vi "Write grouped data to tags.vi"(9 "Indices":i32[](array[numeric]), 10 "Data Type":T1, 11 "Data":T2) -> ()   [LabVIEW 2016, in "CVT.lvlib" / "Current Value Table.lvlib"]
uses:
  <vilib>/NI/Current Value Table/Current Value Table.lvlib
  <vilib>/NI/Current Value Table/Type Defs/Group Data.ctl
  <vilib>/NI/Current Value Table/Type Defs/Data Types.ctl
  <vilib>/NI/Current Value Table/DataTypes/Double_Write Index Set.vi
  <vilib>/NI/Current Value Table/DataTypes/Array of String_Write Index Set.vi
  <vilib>/NI/Current Value Table/DataTypes/Array of Boolean_Write Index Set.vi
  <vilib>/NI/Current Value Table/DataTypes/Array of Single_Write Index Set.vi
  <vilib>/NI/Current Value Table/DataTypes/Array of Double_Write Index Set.vi
  <vilib>/NI/Current Value Table/DataTypes/Array of I8_Write Index Set.vi
  <vilib>/NI/Current Value Table/DataTypes/Array of I16_Write Index Set.vi
  <vilib>/NI/Current Value Table/DataTypes/Array of I32_Write Index Set.vi
  <vilib>/NI/Current Value Table/DataTypes/Array of I64_Write Index Set.vi
  <vilib>/NI/Current Value Table/DataTypes/Array of U64_Write Index Set.vi
  <vilib>/NI/Current Value Table/DataTypes/Array of U32_Write Index Set.vi
  <vilib>/NI/Current Value Table/DataTypes/Array of U16_Write Index Set.vi
  <vilib>/NI/Current Value Table/DataTypes/Array of U8_Write Index Set.vi
  <vilib>/NI/Current Value Table/DataTypes/Boolean_Write Index Set.vi
  <vilib>/NI/Current Value Table/DataTypes/String_Write Index Set.vi
  <vilib>/NI/Current Value Table/DataTypes/U8_Write Index Set.vi
  <vilib>/NI/Current Value Table/DataTypes/U16_Write Index Set.vi
  <vilib>/NI/Current Value Table/DataTypes/U32_Write Index Set.vi
  <vilib>/NI/Current Value Table/DataTypes/U64_Write Index Set.vi
  <vilib>/NI/Current Value Table/DataTypes/I8_Write Index Set.vi
  <vilib>/NI/Current Value Table/DataTypes/I16_Write Index Set.vi
  <vilib>/NI/Current Value Table/DataTypes/I32_Write Index Set.vi
  <vilib>/NI/Current Value Table/DataTypes/I64_Write Index Set.vi
  <vilib>/NI/Current Value Table/DataTypes/Single_Write Index Set.vi
  <vilib>/NI/Current Value Table/Memory Block.vi
  <vilib>/NI/Current Value Table/DataTypes/Single_Memory Block.vi
  <vilib>/NI/Current Value Table/DataTypes/I64_Memory Block.vi
  <vilib>/NI/Current Value Table/DataTypes/I32_Memory Block.vi
  <vilib>/NI/Current Value Table/DataTypes/I16_Memory Block.vi
  <vilib>/NI/Current Value Table/DataTypes/I8_Memory Block.vi
  <vilib>/NI/Current Value Table/DataTypes/U64_Memory Block.vi
  <vilib>/NI/Current Value Table/DataTypes/U32_Memory Block.vi
  <vilib>/NI/Current Value Table/DataTypes/U16_Memory Block.vi
  <vilib>/NI/Current Value Table/DataTypes/U8_Memory Block.vi
  <vilib>/NI/Current Value Table/DataTypes/String_Memory Block.vi
  <vilib>/NI/Current Value Table/DataTypes/Boolean_Memory Block.vi
  <vilib>/NI/Current Value Table/DataTypes/Array of U8_Memory Block.vi
  <vilib>/NI/Current Value Table/DataTypes/Array of U16_Memory Block.vi
  <vilib>/NI/Current Value Table/DataTypes/Array of U32_Memory Block.vi
  <vilib>/NI/Current Value Table/DataTypes/Array of U64_Memory Block.vi
  <vilib>/NI/Current Value Table/DataTypes/Array of I64_Memory Block.vi
  <vilib>/NI/Current Value Table/DataTypes/Array of I32_Memory Block.vi
  <vilib>/NI/Current Value Table/DataTypes/Array of I16_Memory Block.vi
  <vilib>/NI/Current Value Table/DataTypes/Array of I8_Memory Block.vi
  <vilib>/NI/Current Value Table/DataTypes/Array of Double_Memory Block.vi
  <vilib>/NI/Current Value Table/DataTypes/Array of Single_Memory Block.vi
  <vilib>/NI/Current Value Table/DataTypes/Array of Boolean_Memory Block.vi
  <vilib>/NI/Current Value Table/DataTypes/Array of String_Memory Block.vi
  <vilib>/NI/Current Value Table/DataTypes/Double_Memory Block.vi
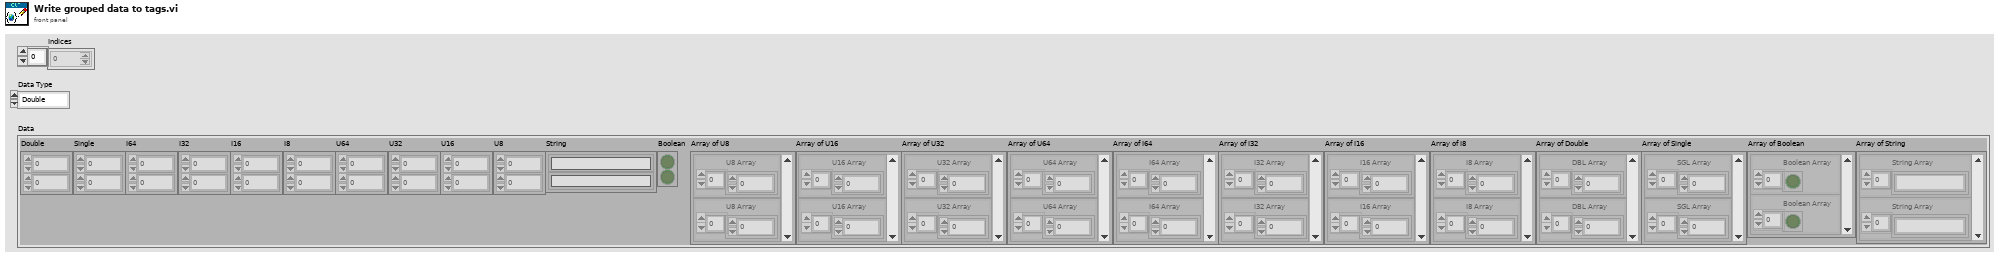
[diagram p1: front panel]
types:
  T1 = typedef "CVT.lvlib/Current Value Table.lvlib/Data Types.ctl" = enum16{"Double", "Single", "I64", "I32", "I16", "I8", "U64", "U32", "U16", "U8", "String", "Boolean", "Array of U8", "Array of U16", "Array of U32", "Array of U64", "Array of I64", "Array of I32", "Array of I16", "Array of I8", "Array of Double", "Array of Single", "Array of Boolean", "Array of String"}
  T2 = typedef "CVT.lvlib/Current Value Table.lvlib/Group Data.ctl" = cluster{"Double":dbl[], "Single":sgl[], "I64":i64[], "I32":i32[], "I16":i16[], "I8":i8[], "U64":u64[], "U32":u32[], "U16":u16[], "U8":u8[], "String":string[], "Boolean":bool[], "Array of U8":cluster{"U8 Array":u8[]}[], "Array of U16":cluster{"U16 Array":u16[]}[], "Array of U32":cluster{"U32 Array":u32[]}[], "Array of U64":cluster{"U64 Array":u64[]}[], "Array of I64":cluster{"I64 Array":i64[]}[], "Array of I32":cluster{"I32 Array":i32[]}[], "Array of I16":cluster{"I16 Array":i16[]}[], "Array of I8":cluster{"I8 Array":i8[]}[], "Array of Double":cluster{"DBL Array":dbl[]}[], "Array of Single":cluster{"SGL Array":sgl[]}[], "Array of Boolean":cluster{"Boolean Array":bool[]}[], "Array of String":cluster{"String Array":string[]}[]}
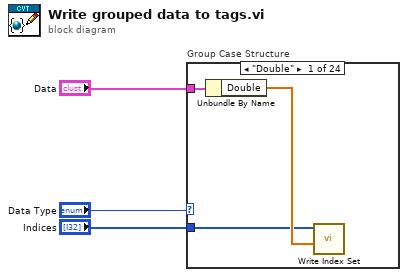
[diagram p0: block diagram]
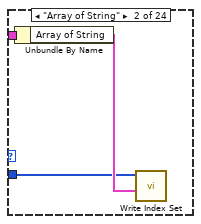
[diagram p2: hidden frame]
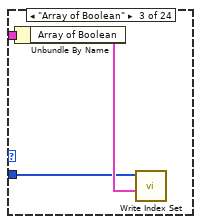
[diagram p3: hidden frame]
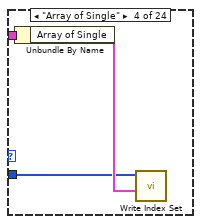
[diagram p4: hidden frame]
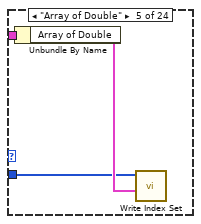
[diagram p5: hidden frame]
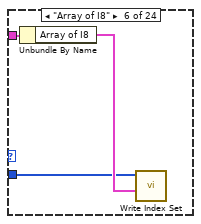
[diagram p6: hidden frame]
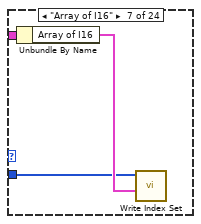
[diagram p7: hidden frame]
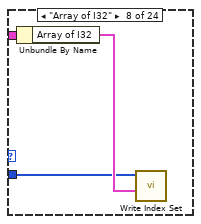
[diagram p8: hidden frame]
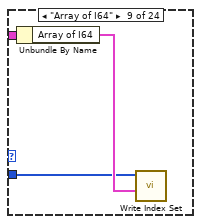
[diagram p9: hidden frame]
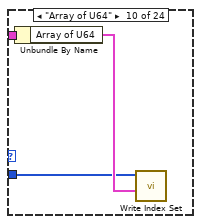
[diagram p10: hidden frame]
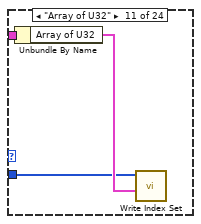
[diagram p11: hidden frame]
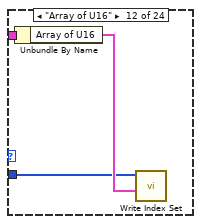
[diagram p12: hidden frame]
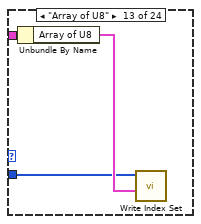
[diagram p13: hidden frame]
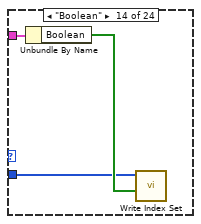
[diagram p14: hidden frame]
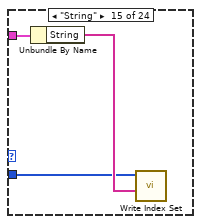
[diagram p15: hidden frame]
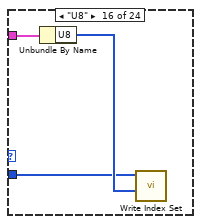
[diagram p16: hidden frame]
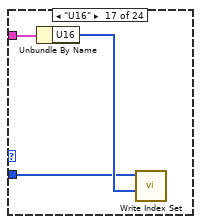
[diagram p17: hidden frame]
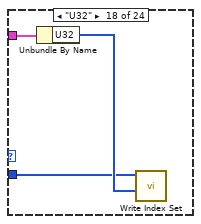
[diagram p18: hidden frame]
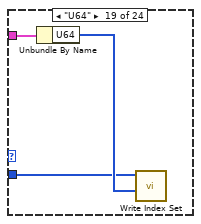
[diagram p19: hidden frame]
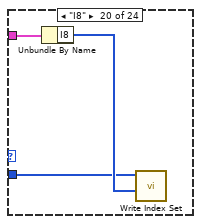
[diagram p20: hidden frame]
diagram:
  n1 = case "Group Case Structure" shown="\"Double\"" "Data Type" {
    tunnel: "Data" -> [w6 w9 w12 w15 w18 w21 w24 w27 w30 w33 w36 w39 w42 w45 w48 w51 w54 w57 w60 w63 w66 w69 w72 w75]
    tunnel: "Indices" -> [w4 w7 w10 w13 w16 w19 w22 w25 w28 w31 w34 w37 w40 w43 w46 w49 w52 w55 w58 w61 w64 w67 w70 w73]
    frame "Double" {
      n2 = Unbundle By Name(w6) -> ("Double"=w5:dbl[])
      n3 = call-poly <vilib>:"Write Index Set.vi"("Values"=w5, "Indices"=w4) -> ()  [unwired: 10 in]
    }
    frame "Array of String" {
      n4 = Unbundle By Name(w9) -> ("Array of String"=w8:cluster{"String Array":string[]}[])
      n5 = call-poly <vilib>:"Write Index Set.vi"("Values"=w8, "Indices"=w7) -> ()  [unwired: 10 in]
    }
    frame "Array of Boolean" {
      n6 = Unbundle By Name(w12) -> ("Array of Boolean"=w11:cluster{"Boolean Array":bool[]}[])
      n7 = call-poly <vilib>:"Write Index Set.vi"("Values"=w11, "Indices"=w10) -> ()  [unwired: 10 in]
    }
    frame "Array of Single" {
      n8 = Unbundle By Name(w15) -> ("Array of Single"=w14:cluster{"SGL Array":sgl[]}[])
      n9 = call-poly <vilib>:"Write Index Set.vi"("Values"=w14, "Indices"=w13) -> ()  [unwired: 10 in]
    }
    frame "Array of Double" {
      n10 = Unbundle By Name(w18) -> ("Array of Double"=w17:cluster{"DBL Array":dbl[]}[])
      n11 = call-poly <vilib>:"Write Index Set.vi"("Values"=w17, "Indices"=w16) -> ()  [unwired: 10 in]
    }
    frame "Array of I8" {
      n12 = Unbundle By Name(w21) -> ("Array of I8"=w20:cluster{"I8 Array":i8[]}[])
      n13 = call-poly <vilib>:"Write Index Set.vi"("Values"=w20, "Indices"=w19) -> ()  [unwired: 10 in]
    }
    frame "Array of I16" {
      n14 = Unbundle By Name(w24) -> ("Array of I16"=w23:cluster{"I16 Array":i16[]}[])
      n15 = call-poly <vilib>:"Write Index Set.vi"("Values"=w23, "Indices"=w22) -> ()  [unwired: 10 in]
    }
    frame "Array of I32" {
      n16 = Unbundle By Name(w27) -> ("Array of I32"=w26:cluster{"I32 Array":i32[]}[])
      n17 = call-poly <vilib>:"Write Index Set.vi"("Values"=w26, "Indices"=w25) -> ()  [unwired: 10 in]
    }
    frame "Array of I64" {
      n18 = Unbundle By Name(w30) -> ("Array of I64"=w29:cluster{"I64 Array":i64[]}[])
      n19 = call-poly <vilib>:"Write Index Set.vi"("Values"=w29, "Indices"=w28) -> ()  [unwired: 10 in]
    }
    frame "Array of U64" {
      n20 = Unbundle By Name(w33) -> ("Array of U64"=w32:cluster{"U64 Array":u64[]}[])
      n21 = call-poly <vilib>:"Write Index Set.vi"("Values"=w32, "Indices"=w31) -> ()  [unwired: 10 in]
    }
    frame "Array of U32" {
      n22 = Unbundle By Name(w36) -> ("Array of U32"=w35:cluster{"U32 Array":u32[]}[])
      n23 = call-poly <vilib>:"Write Index Set.vi"("Values"=w35, "Indices"=w34) -> ()  [unwired: 10 in]
    }
    frame "Array of U16" {
      n24 = Unbundle By Name(w39) -> ("Array of U16"=w38:cluster{"U16 Array":u16[]}[])
      n25 = call-poly <vilib>:"Write Index Set.vi"("Values"=w38, "Indices"=w37) -> ()  [unwired: 10 in]
    }
    frame "Array of U8" {
      n26 = Unbundle By Name(w42) -> ("Array of U8"=w41:cluster{"U8 Array":u8[]}[])
      n27 = call-poly <vilib>:"Write Index Set.vi"("Values"=w41, "Indices"=w40) -> ()  [unwired: 10 in]
    }
    frame "Boolean" {
      n28 = Unbundle By Name(w45) -> ("Boolean"=w44:bool[])
      n29 = call-poly <vilib>:"Write Index Set.vi"("Values"=w44, "Indices"=w43) -> ()  [unwired: 10 in]
    }
    frame "String" {
      n30 = Unbundle By Name(w48) -> ("String"=w47:string[])
      n31 = call-poly <vilib>:"Write Index Set.vi"("Values"=w47, "Indices"=w46) -> ()  [unwired: 10 in]
    }
    frame "U8" {
      n32 = Unbundle By Name(w51) -> ("U8"=w50:u8[])
      n33 = call-poly <vilib>:"Write Index Set.vi"("Values"=w50, "Indices"=w49) -> ()  [unwired: 10 in]
    }
    frame "U16" {
      n34 = Unbundle By Name(w54) -> ("U16"=w53:u16[])
      n35 = call-poly <vilib>:"Write Index Set.vi"("Values"=w53, "Indices"=w52) -> ()  [unwired: 10 in]
    }
    frame "U32" {
      n36 = Unbundle By Name(w57) -> ("U32"=w56:u32[])
      n37 = call-poly <vilib>:"Write Index Set.vi"("Values"=w56, "Indices"=w55) -> ()  [unwired: 10 in]
    }
    frame "U64" {
      n38 = Unbundle By Name(w60) -> ("U64"=w59:u64[])
      n39 = call-poly <vilib>:"Write Index Set.vi"("Values"=w59, "Indices"=w58) -> ()  [unwired: 10 in]
    }
    frame "I8" {
      n40 = Unbundle By Name(w63) -> ("I8"=w62:i8[])
      n41 = call-poly <vilib>:"Write Index Set.vi"("Values"=w62, "Indices"=w61) -> ()  [unwired: 10 in]
    }
    frame "I16" {
      n42 = Unbundle By Name(w66) -> ("I16"=w65:i16[])
      n43 = call-poly <vilib>:"Write Index Set.vi"("Values"=w65, "Indices"=w64) -> ()  [unwired: 10 in]
    }
    frame "I32" {
      n44 = Unbundle By Name(w69) -> ("I32"=w68:i32[])
      n45 = call-poly <vilib>:"Write Index Set.vi"("Values"=w68, "Indices"=w67) -> ()  [unwired: 10 in]
    }
    frame "I64" {
      n46 = Unbundle By Name(w72) -> ("I64"=w71:i64[])
      n47 = call-poly <vilib>:"Write Index Set.vi"("Values"=w71, "Indices"=w70) -> ()  [unwired: 10 in]
    }
    frame "Single" {
      n48 = Unbundle By Name(w75) -> ("Single"=w74:sgl[])
      n49 = call-poly <vilib>:"Write Index Set.vi"("Values"=w74, "Indices"=w73) -> ()  [unwired: 10 in]
    }
  }
